vi "Read All Channels.vi"(8 "error in":errorcluster, 11 "DI DAQmx Cont CFG in":refnum<class "DI DAQmx Cont CFG.lvclass">) -> (0 "error out":errorcluster, 2 "Readings":variant, 3 "DI DAQmx Cont CFG out":refnum<class "DI DAQmx Cont CFG.lvclass">)   [LabVIEW 2024, in "DI DAQmx Cont CFG.lvclass"]
uses:
  DI DAQmx Cont CFG.lvclass
  DI DAQmx Cont CFG.lvclass/DI DAQmx Cont CFG.ctl
  Buffers/Buffer Lossless Digital/Buffer Lossless Digital.lvclass
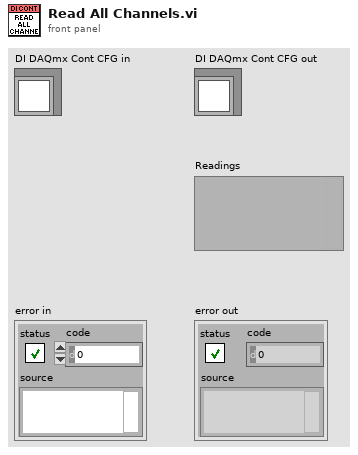
[diagram p1: front panel]
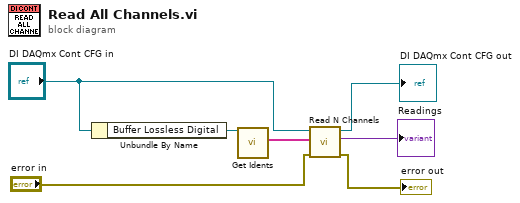
[diagram p0: block diagram]
diagram:
  n1 = Unbundle By Name("DI DAQmx Cont CFG in") -> ("Buffer Lossless Digital"=w7:refnum<class "Buffer Lossless Digital.lvclass">)
  n2 = call "Get Idents.vi"("Buffer Lossless Digital in"=w7) -> ("Idents"=w6:string[])  [unwired: 9 in, 1 out]
  n3 = call-dynamic "Read N Channels.vi"("error in"="error in", "Channels"=w6, "DI DAQmx Cont CFG in"="DI DAQmx Cont CFG in") -> ("error out"=→"error out":errorcluster, "Readings"=→"Readings":variant, "DI DAQmx Cont CFG out"=→"DI DAQmx Cont CFG out":refnum<class "DI DAQmx Cont CFG.lvclass">)  [unwired: 6 in]
